vi "Active Noise Control with Feedback Neutralization (RT).vi"() -> ()   [LabVIEW 2019]
doc: "This VI runs on an RT target. This VI downloads the Active Noise Control with Feedback Neutralization (FPGA) VI to FPGA, estimates the coefficients of the feedback path and secondary path, runs the Active Noise Control with Feedback Neutralization (FPGA) VI on FPGA, communicates with the Active Noise Control with Feedback Neutralization (FPGA) VI to read and display the residual noise at the location of interest. \n\nComplete the following steps to use this example.\n\n1. Run this VI.\n\n2. Configure the settings for the feedback path and secondary path modeling in the <b>Feedback Path and Secondary Path Modeling</b> page.\n\n3. Click the <b>Start</b> button to estimate the coefficients of feedback path and secondary path. This VI uses LMS adaptive filters to estimate the coefficients.\n\n4. Click the <b>Next</b> button to display the <b>Active Noise Control</b> page.\n\n5. Configure the step size of the filtered-X LMS adaptive filter in the <b>Active Noise Control</b> page. The filter length of the filtered-X LMS adaptive filter is the same as <b>Filter Length</b> in the <b>Feedback Path and Secondary Path Modeling</b> page.\n \n6. Enable the <b>Control on</b> option. Verify whether the noise is reduced.\n\n7. Click the <b>Stop</b> button to stop this VI."
uses:
  <vilib>/userdefined/High Color/nirio_resource_hc.ctl
  <vilib>/FPGAPlugInAG/cRIO-9033/niLvFpga_Open_cRIO-9033.vi
  <vilib>/addons/Adaptive Filters/Create/AFT Create FIR LMS (Real).vi
  <vilib>/Utility/error.llb/Error Cluster From Error Code.vi
  <vilib>/rvi/errors/niLvFpgaAdjustHostInterfaceError.vi
  <vilib>/FPGAPlugInAG/cRIO-9033/niLvFpga_Run_cRIO-9033.vi
  <vilib>/addons/Adaptive Filters/Processing/AFT Filter Signal and Update Coefficients (Real, Array).vi
  <vilib>/addons/Adaptive Filters/Analysis/AFT Get Coefficients (FIR, Real).vi
  <vilib>/FPGAPlugInAG/cRIO-9033/niLvFpga_Close_cRIO-9033.vi
  <vilib>/rvi/interface/nirviOpenFPGA/nirviOpenFPGA.xnode
  FPGA Bitfiles/activenoisecontr_FPGATarget_ActiveNoiseContr_mCFUFk62OtE.lvbitx
  Active Noise Control with Feedback Neutralization (FPGA).vi
  <vilib>/rvi/interface/nirviReadWriteControl/nirviReadWriteControl.xnode
  <vilib>/rvi/interface/nirviMethod/nirviMethod.xnode
  <vilib>/rvi/interface/nirviCloseFPGA/nirviCloseFPGA.xnode
  <vilib>/addons/Adaptive Filters/NI_AdaptiveFilter.lvlib
  <vilib>/rvi/errors/niLvFpgaMergeErrorWithErrorCode.vi
  NiFpgaLv.dll
  <vilib>/FPGAPlugInAG/cRIO-9033/niLvFpga_ReadFifo_cRIO-9033.vi
  <vilib>/FPGAPlugInAG/cRIO-9033/niLvFpga_WriteFifo_cRIO-9033.vi
panel:
  in  "Tab Control":T1(tab)=enum."Feedback Path and Secondary Path Modeling"
  in  "Next":bool
  in  "Step Size (LMS)":dbl=0.002
  in  "Filter Length":i32=300 format="%#.0f"
  in  "Start":bool
  out "Secondary Path Coefficients":dbl[](graph)
  out "Feedback Path Coefficients":dbl[](graph)
  in  "RIO Device":T2="RIO0"
  in  "Control on":bool
  out "Power Spectrum of Residual Noise":cluster{"f0":dbl, "df":dbl, "magnitude":dbl[]}(graph)
  out "Residual Noise":dbl[](graph)
  in  "Reset":bool
  in  "Stop":bool
  in  "step size":dbl=0.002 caption="Step Size (FXLMS)"
  # "Active Noise Control with Feedback Neutralization"
  # "Refer to the Active Noise Control topic in the LabVIEW Help for more information about the background of active noise control. Select Help>>Show Context Help and move the cursor over the VI icon of this example for more information."
  # "Feedback Path and Secondary Path Modeling"
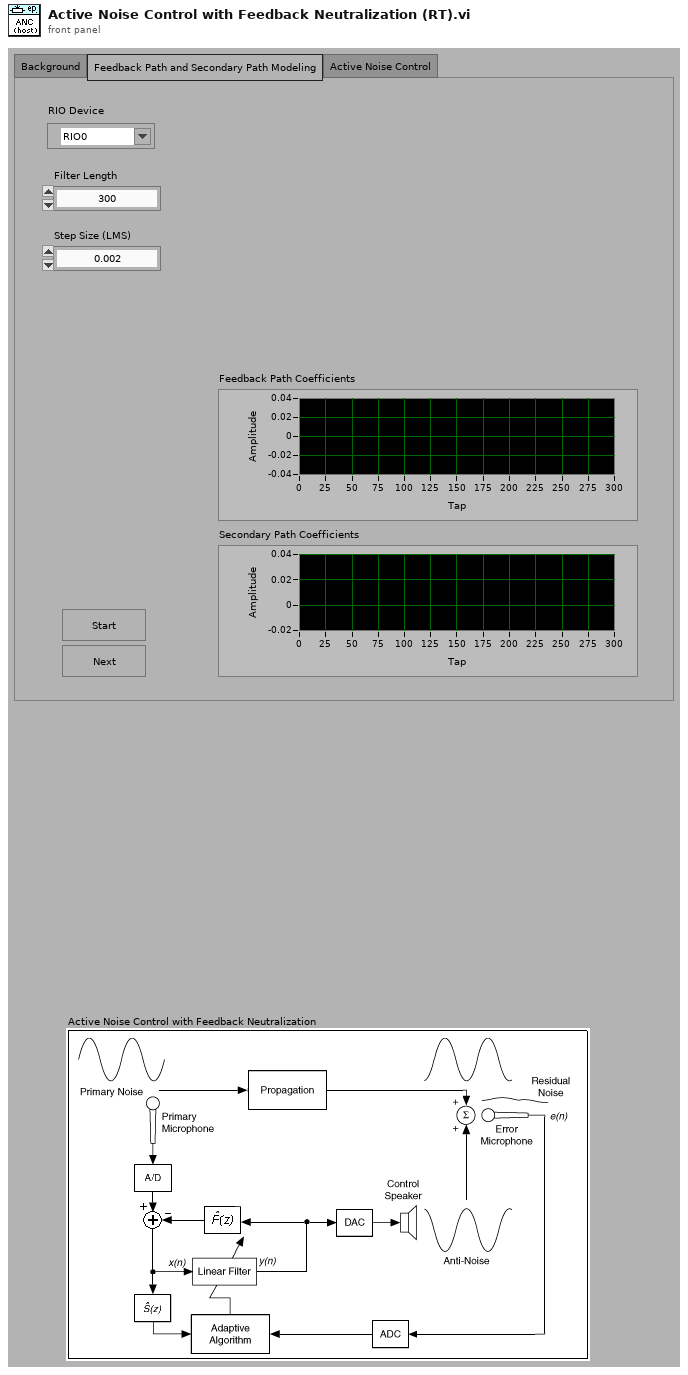
[diagram p1: front panel]
types:
  T1 = enum32{"Background", "Feedback Path and Secondary Path Modeling", "Active Noise Control"}
  T2 = typedef "nirio_resource_hc.ctl" = tag
  T3 = enum8{"Enabled", "Disabled", "Disabled and Grayed Out"}
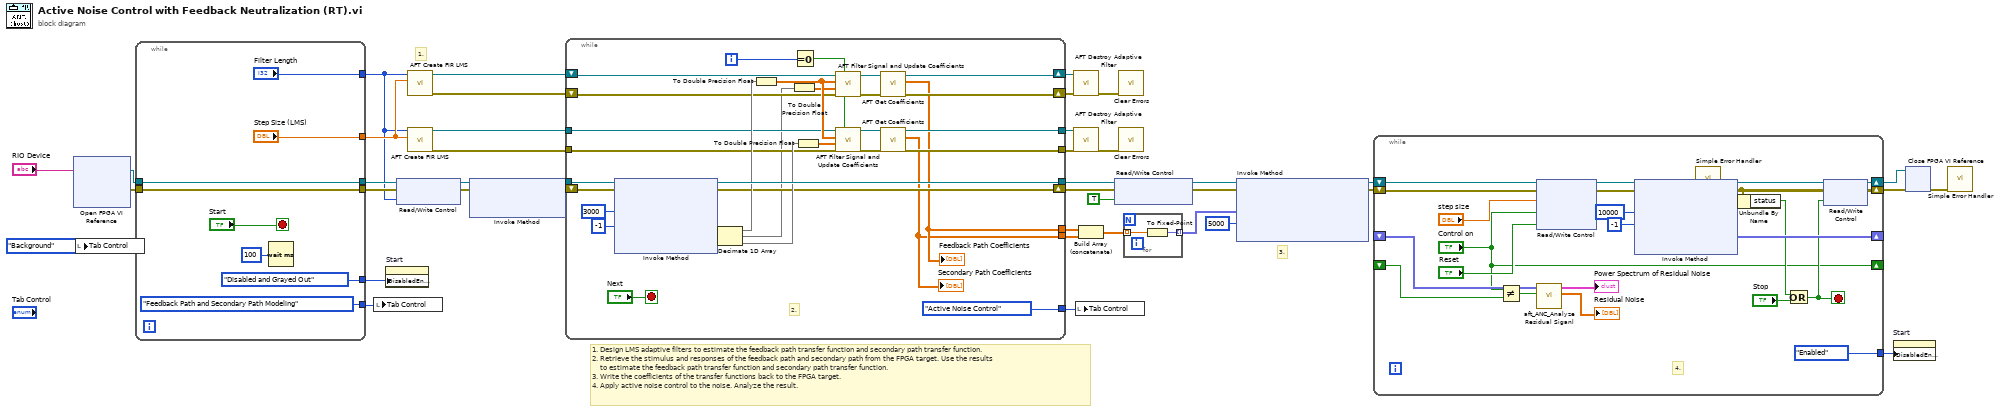
[diagram p0: block diagram]
diagram:
  # "3."
  # "1."
  # "1. Design LMS adaptive filters to estimate the feedback path transfer function and secondary path transfer function.\n2. Retrieve the stimulus and responses of the feedback path and secondary path from the FPGA target. Use the results \n    to estimate the feedback path transfer function and secondary path transfer function.\n3. Write the coefficients of the transfer functions back to the FPGA target.\n4. Apply active noise control to the noise. Analyze the result."
  n1 = xnode "Open FPGA VI Reference"("resource name"="RIO Device") -> ("FPGA VI Reference Out"=w10:refnum<k20>, "error out"=w11:errorcluster)  [unwired: 1 in]
  n2 = local write "Tab Control"(T1."Background" ("Tab Control")) -> ()
  n3 = while {
    tunnel: w11 -> [w48]
    tunnel: w10 -> [w47]
    tunnel: [w48] -> w22
    tunnel: [w47] -> w20
    tunnel: ["Filter Length"] -> w18
    tunnel: ["Step Size (LMS)"] -> w23
    tunnel: [T3."Disabled and Grayed Out" ("Disabled")] -> w17
    tunnel: [T1."Feedback Path and Secondary Path Modeling" ("Tab Control")] -> w5
    stop <- "Start" stop-if-true
    n4 = Wait (ms)(milliseconds to wait=u32 100) -> ()  [unwired: 1 out]
  }
  n5 = local write "Tab Control"(w5) -> ()
  n6 = property on="Start" class="Bool"("DisabledEnum"=w17) -> ()  [unwired: 2 in, 2 out]
  n7 = xnode "Read/Write Control"("FPGA VI Reference In"=w20, "error in"=w22, "filter length"=w18) -> ("FPGA VI Reference Out"=w19:refnum<k20>, "error out"=w21:errorcluster)
  n8 = call-poly <vilib>:"AFT Create FIR LMS.vi"("step size"=w23, "filter length"=w18) -> ("error out"=w33:errorcluster, "adaptive filter out"=w15:refnum<k20>)  [unwired: 2 in, 6 out]
  n9 = call-poly <vilib>:"AFT Create FIR LMS.vi"("step size"=w23, "filter length"=w18) -> ("error out"=w32:errorcluster, "adaptive filter out"=w14:refnum<k20>)  [unwired: 2 in, 6 out]
  n10 = xnode "Invoke Method"("FPGA VI Reference In"=w19, "error in"=w21) -> ("FPGA VI Reference Out"=w27:refnum<k20>, "error out"=w28:errorcluster)  [unwired: 1 in]
  n11 = while {
    tunnel: w27 -> [w77]
    shift-right: [w56] -> w26
    shift-left: w28 -> [w79]
    tunnel: [w55] -> w3
    tunnel: [w54] -> w2
    tunnel: [w76] -> w9
    tunnel: w32 -> [w61]
    tunnel: [w57] -> w30
    tunnel: w14 -> [w62]
    tunnel: [w58] -> w12
    shift-right: [w60] -> w29
    shift-left: w33 -> [w63]
    shift-right: [w59] -> w13
    shift-left: w15 -> [w64]
    tunnel: [T1."Active Noise Control" ("Tab Control")] -> w4
    i -> [w53]
    stop <- "Next" stop-if-true
    # "2."
    n12 = xnode "Invoke Method"("FPGA VI Reference In"=w77, "error in"=w79, "Number of Elements"=u32 3000 ("#samples"), "Timeout (ms)"=-1) -> ("FPGA VI Reference Out"=w76:refnum<k20>, "error out"=w56:errorcluster, "Data"=w65:fxp<+/-,24,4>[])  [unwired: 1 out]
    n13 = Decimate 1D Array(w65) -> (w70:fxp<+/-,24,4>[], w50:fxp<+/-,24,4>[], w68:fxp<+/-,24,4>[])
    n14 = To Double Precision Float(number=w70) -> (double precision float=w69:dbl[])
    n15 = To Double Precision Float(number=w50) -> (double precision float=w67:dbl[])
    n16 = Equal To 0?(x=w53) -> (x = 0?=w52:bool)
    n17 = To Double Precision Float(number=w68) -> (double precision float=w66:dbl[])
    n18 = call-poly <vilib>:"AFT Filter Signal and Update Coefficients.vi"("reset? (F)"=w52, "error in (no error)"=w63, "d(n)"=w67, "x(n)"=w69, "adaptive filter in"=w64) -> ("error out"=w73:errorcluster, "adaptive filter out"=w74:refnum<k20>)  [unwired: 1 in, 4 out]
    n19 = call-poly <vilib>:"AFT Filter Signal and Update Coefficients.vi"("reset? (F)"=w52, "error in (no error)"=w61, "d(n)"=w66, "x(n)"=w69, "adaptive filter in"=w62) -> ("error out"=w71:errorcluster, "adaptive filter out"=w72:refnum<k20>)  [unwired: 1 in, 4 out]
    n20 = call-poly <vilib>:"AFT Get Coefficients.vi"("error in (no error)"=w73, "adaptive filter in"=w74) -> ("error out"=w60:errorcluster, "coefficients"=w55:dbl[], "adaptive filter out"=w59:refnum<k20>)  [unwired: 7 in]
    "Feedback Path Coefficients" <- w55
    n21 = call-poly <vilib>:"AFT Get Coefficients.vi"("error in (no error)"=w71, "adaptive filter in"=w72) -> ("error out"=w57:errorcluster, "coefficients"=w54:dbl[], "adaptive filter out"=w58:refnum<k20>)  [unwired: 7 in]
    "Secondary Path Coefficients" <- w54
  }
  n22 = call <vilib>:"AFT Destroy Adaptive Filter.vi"("error in (no error)"=w29, "adaptive filter in"=w13) -> ("error out"=w34:errorcluster)  [unwired: 9 in]
  n23 = call <vilib>:"AFT Destroy Adaptive Filter.vi"("error in (no error)"=w30, "adaptive filter in"=w12) -> ("error out"=w31:errorcluster)  [unwired: 9 in]
  n24 = local write "Tab Control"(w4) -> ()
  n25 = Build Array (concatenate)(w3, w2) -> (w39:dbl[])
  n26 = xnode "Read/Write Control"("FPGA VI Reference In"=w9, "error in"=w26, "stop modeling"=TRUE) -> ("FPGA VI Reference Out"=w8:refnum<k20>, "error out"=w25:errorcluster)
  n27 = call <vilib>:"Clear Errors.vi"("error in (no error)"=w34) -> ()  [unwired: 5 in, 2 out]
  n28 = call <vilib>:"Clear Errors.vi"("error in (no error)"=w31) -> ()  [unwired: 5 in, 2 out]
  n29 = for {
    tunnel: w39 -> [w82] mode=indexing
    tunnel: [w81] -> w38 mode=indexing
    n30 = To Fixed-Point(number=w82) -> (fixed-point=w81:fxp<+/-,32,4>)  [unwired: 1 in]
  }
  n31 = xnode "Invoke Method"("FPGA VI Reference In"=w8, "error in"=w25, "Data"=w38, "Timeout (ms)"=5000) -> ("FPGA VI Reference Out"=w6:refnum<k20>, "error out"=w7:errorcluster)  [unwired: 1 out]
  n32 = while {
    shift-right: [w99] -> _
    shift-left: _ -> [w92]
    shift-right: [w101] -> w36
    shift-left: w7 -> [w104]
    shift-right: [w102] -> w37
    shift-left: w6 -> [w105]
    shift-right: ["Control on"] -> _
    shift-left: _ -> [w98]
    tunnel: [T3."Enabled" ("Disabled")] -> w16
    stop <- w88 stop-if-true
    # "4."
    n33 = Not Equal?(x="Control on", y=w98) -> (x != y?=w91:bool)
    n34 = xnode "Read/Write Control"("FPGA VI Reference In"=w105, "error in"=w104, "step size"="step size", "control on"="Control on", "reset? (F)"="Reset") -> ("FPGA VI Reference Out"=w95:refnum<k20>, "error out"=w94:errorcluster)
    n35 = call "aft_ANC_Analyze Residual Siganl.vi"("restart averaging"=w91, "signal"=w92) -> ("residual noise"=→"Residual Noise":dbl[], "power spectrum"=→"Power Spectrum of Residual Noise":cluster{"f0":dbl, "df":dbl, "magnitude":dbl[]})  [unwired: 8 in]
    n36 = xnode "Invoke Method"("FPGA VI Reference In"=w95, "error in"=w94, "Number of Elements"=u32 10000, "Timeout (ms)"=-1) -> ("FPGA VI Reference Out"=w103:refnum<k20>, "error out"=w93:errorcluster, "Data"=w99:fxp<+/-,24,4>[])  [unwired: 1 out]
    n37 = Unbundle By Name(w93) -> ("status"=w90:bool)
    n38 = Or(x=w90, y="Stop") -> (x .or. y?=w88:bool)
    n39 = xnode "Read/Write Control"("FPGA VI Reference In"=w103, "error in"=w93, "stop"=w88) -> ("FPGA VI Reference Out"=w102:refnum<k20>, "error out"=w101:errorcluster)
  }
  n40 = property on="Start" class="Bool"("DisabledEnum"=w16) -> ()  [unwired: 2 in, 2 out]
  n41 = xnode "Close FPGA VI Reference"("FPGA VI Reference In"=w37, "error in"=w36) -> ("error out"=w35:errorcluster)
  n42 = call <vilib>:"Simple Error Handler.vi"("error in (no error)"=w35) -> ()  [unwired: 1 in, 8 out]
  n43 = call <vilib>:"Simple Error Handler.vi"("error in (no error)"=w35) -> ()  [unwired: 4 in, 5 out]
